vi "AalborgDFCCommand.vi"(4 "Channel Name":string="Aalborg", 6 "Port Name":string="mfc1", 7 "Timeout/ms":u32=1500, 8 "Numeric Value":dbl format="%.2f", 9 "AalborgDFCCommand":T2="FullScaleRatingSLPM", 10 "Address":u8 format="%.0x") -> (0 "String Reply":string="!11,100.0000\r\n", 1 "Error Description":string, 2 "Numeric Reply":dbl=100.0, 3 "OK":bool)   [LabVIEW 2016]
uses:
  AalborgDFCCommand.ctl
  AalborgDFCCommandDescriptor.ctl
  AalborgDFCCommandPhases.ctl
panel:
  out "commandString":string
  out "Audit trail":string[](array[string])
  out "CommandDescriptorOutput":T1={"Command"="FullScaleRatingSLPM", "Mnemonic"="E", "Min"=nan, "Max"=nan, "ActionPath"=["PassCommand", "Communicate", "ParseNumber", "Done"]}
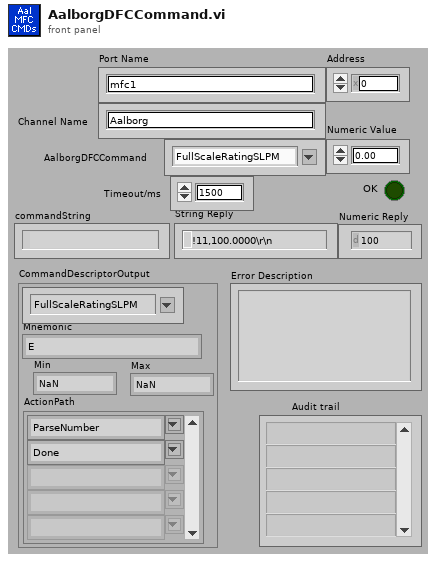
[diagram p1: front panel]
types:
  T1 = typedef "AalborgDFCCommandDescriptor.ctl" = cluster{"Command":T2, "Mnemonic":string, "Min":dbl, "Max":dbl, "ActionPath":T3[]}
  T2 = typedef "AalborgDFCCommand.ctl" = string
  T3 = typedef "AalborgDFCCommandPhases.ctl" = string
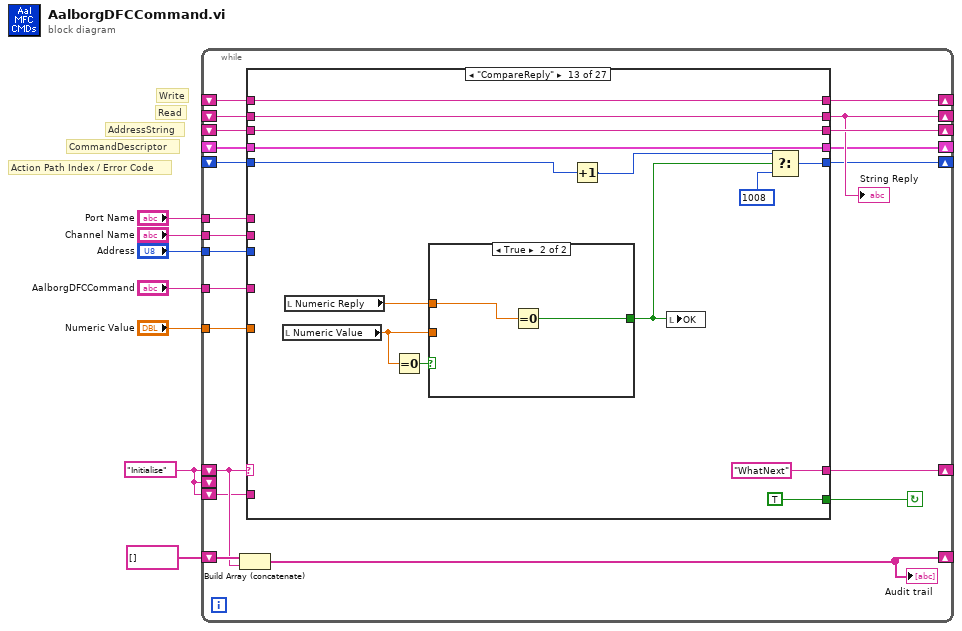
[diagram p0: block diagram]
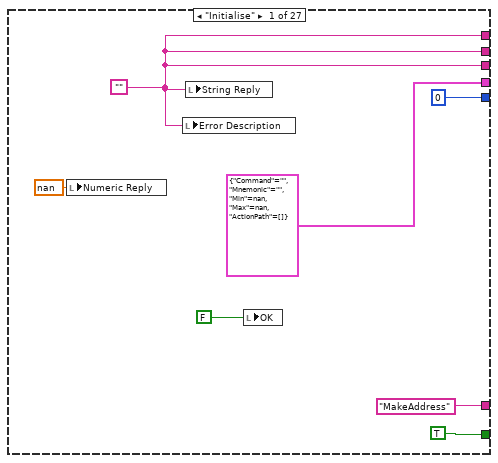
[diagram p2: hidden frame]
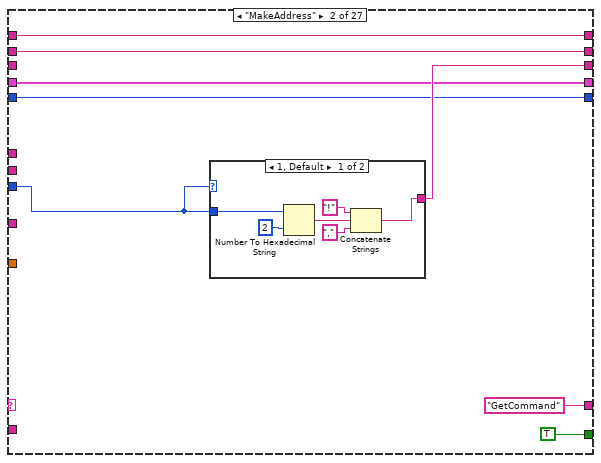
[diagram p3: hidden frame]
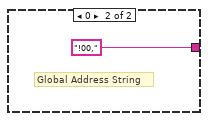
[diagram p4: hidden frame]
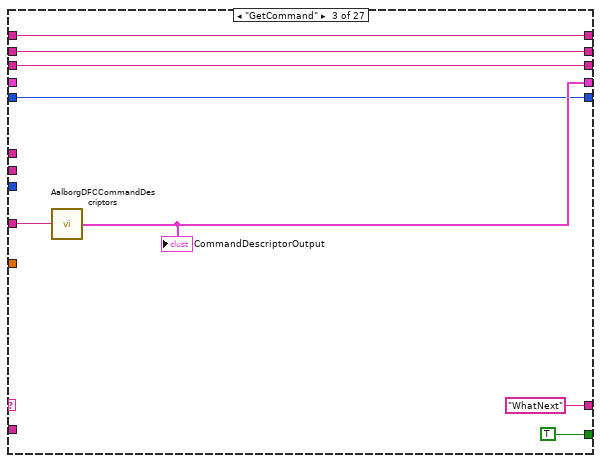
[diagram p5: hidden frame]
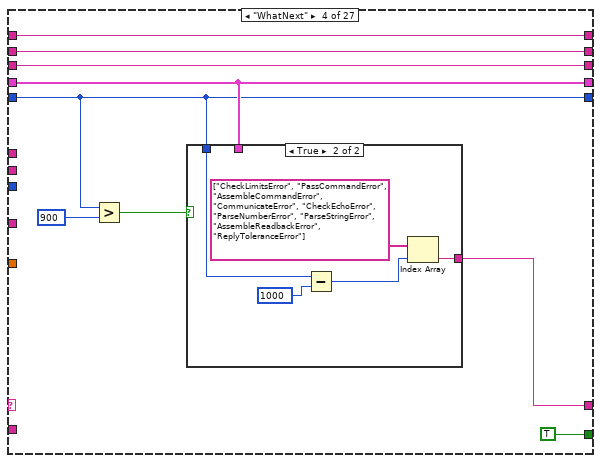
[diagram p6: hidden frame]
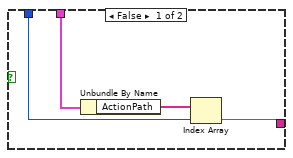
[diagram p7: hidden frame]
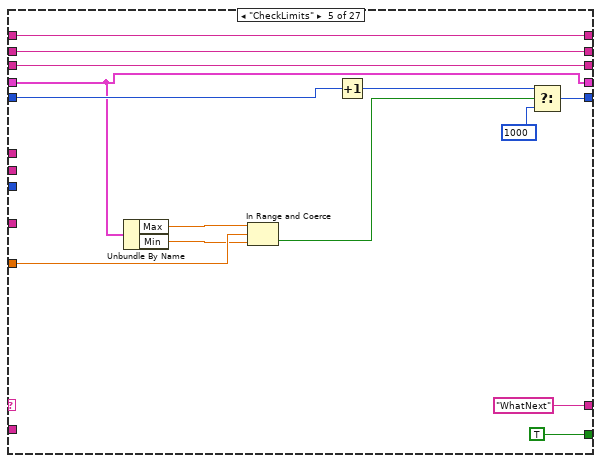
[diagram p8: hidden frame]
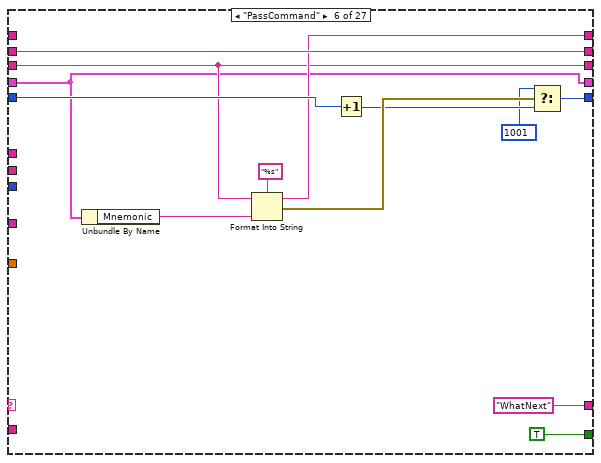
[diagram p9: hidden frame]
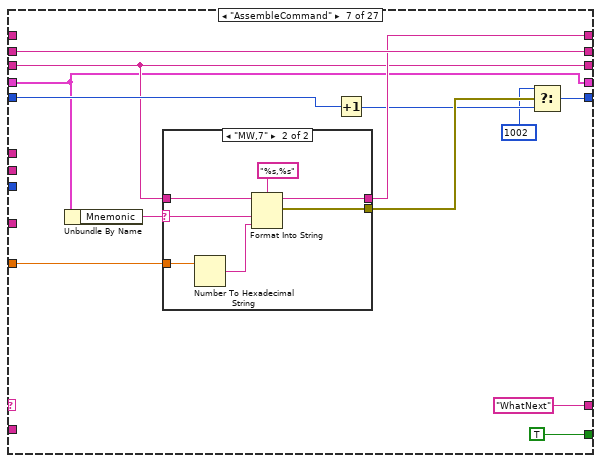
[diagram p10: hidden frame]
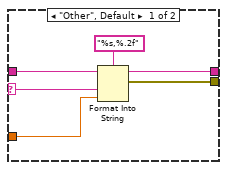
[diagram p11: hidden frame]
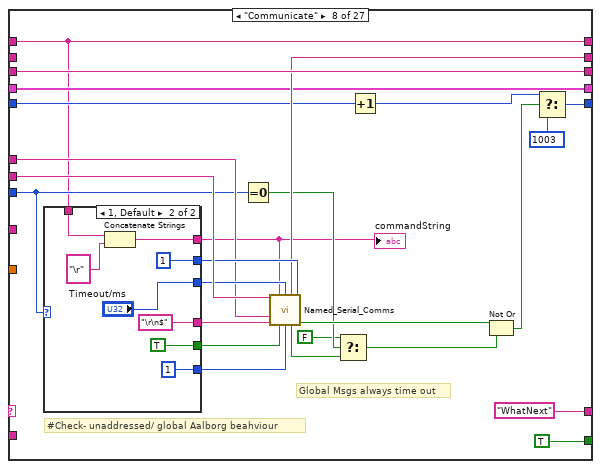
[diagram p12: hidden frame]
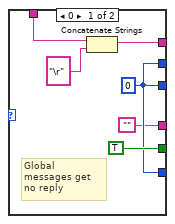
[diagram p13: hidden frame]
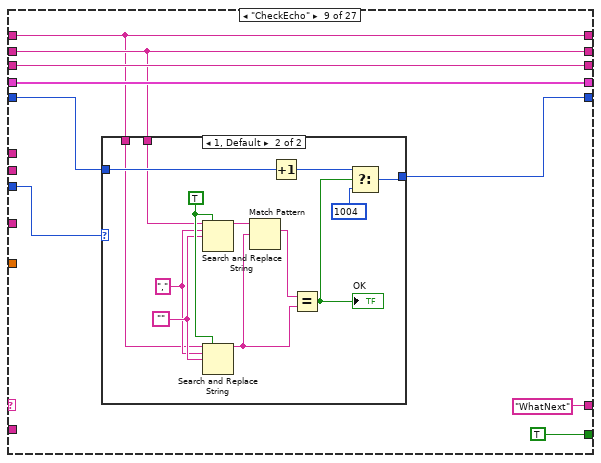
[diagram p14: hidden frame]
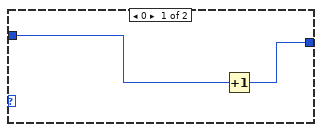
[diagram p15: hidden frame]
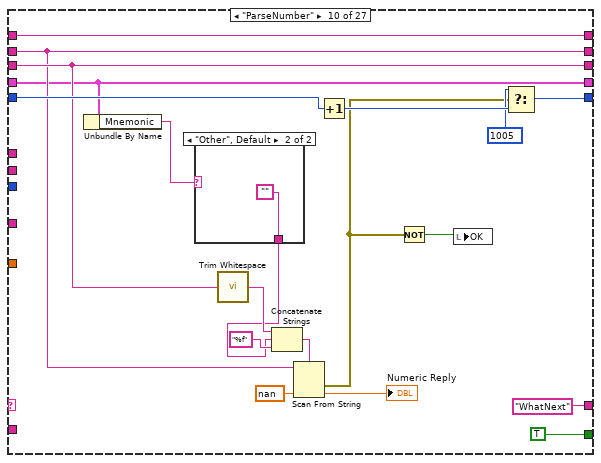
[diagram p16: hidden frame]
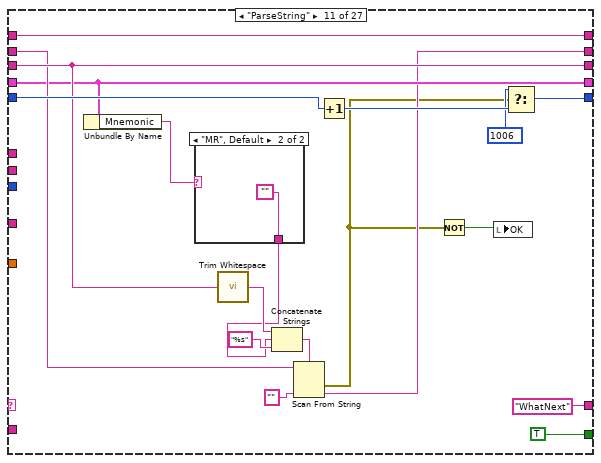
[diagram p18: hidden frame]
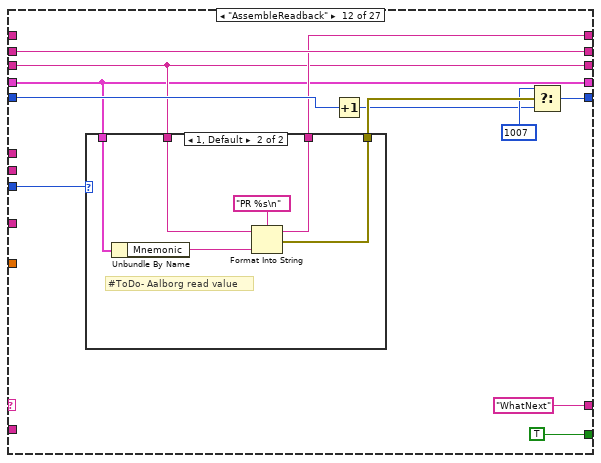
[diagram p20: hidden frame]
diagram:
  w1 = "Initialise"
  # "Action Path Index / Error Code"
  # "CommandDescriptor"
  # "AddressString"
  # "Read"
  # "Write"
  n1 = while {
    shift-right: [w16] -> _
    shift-left: w1 -> [w10]
    tunnel: "Address" -> [w28]
    tunnel: "AalborgDFCCommand" -> [w27]
    tunnel: "Numeric Value" -> [w26]
    shift-right: [w25] -> _
    shift-left: _ -> [w24]
    tunnel: "Port Name" -> [w23]
    tunnel: "Channel Name" -> [w22]
    shift-right: [w15] -> _
    shift-left: _ -> [w21]
    shift-right: [w19] -> _
    shift-left: _ -> [w18]
    shift-right: [w8] -> _
    shift-left: string[] [] -> [w17]
    shift-right: [w14] -> _
    shift-left: _ -> [w13]
    shift-right: [w11] -> _
    shift-left: _ -> [w12]
    shift-left: w1 -> [_]
    shift-left: w1 -> [w9]
    stop <- w20 continue-if-true
    n2 = Build Array (concatenate)(w17, w10) -> (w8:T3[])
    "Audit trail" <- w8
    n3 = case shown="\"CompareReply\"" w10 {
      selector: w10 -> [_ _ _ _ _ _ _ _ _ _ _ _ _ _ _ _ _ _ _ _ _ _ _ _ _ _ w445]
      tunnel: ["MakeAddress" "GetCommand" "WhatNext" w63 "WhatNext" "WhatNext" "WhatNext" "WhatNext" "WhatNext" "WhatNext" "WhatNext" "WhatNext" "WhatNext" w281 "Error" "Initialise" "Error" "Error" "Error" "Error" "Error" "Error" "Error" "Error" "Error" "Error" w445] -> w16
      tunnel: w28 -> [_ w36 _ _ _ _ _ w132 w169 _ _ w238 _ _ _ _ w333 w344 w354 w365 w375 w387 w399 w410 w421 w430 _]
      tunnel: w27 -> [_ _ w55 _ _ _ _ _ _ _ _ _ _ _ _ _ _ _ _ _ _ _ _ _ _ _ _]
      tunnel: w26 -> [_ _ _ _ w88 _ w105 _ _ _ _ _ _ _ _ _ w336 _ w357 _ _ _ _ _ _ _ _]
      tunnel: [w30 w41 w57 w66 w86 w98 w111 w131 w170 w200 w223 w241 w261 w287 w303 w331 w341 w351 w362 w372 w384 w396 w407 w418 w427 w438 w443] -> w25
      tunnel: w24 -> [_ w41 w57 w66 w86 _ _ w131 w170 w200 w223 _ w261 w287 w303 w324 _ _ _ _ w378 w390 _ _ _ _ _]
      tunnel: w23 -> [_ _ _ _ _ _ _ w148 _ _ _ _ _ _ _ w325 _ _ _ _ _ _ _ _ _ _ _]
      tunnel: w22 -> [_ _ _ _ _ _ _ w154 _ _ _ _ _ _ w298 w326 _ _ _ _ _ _ _ _ _ _ _]
      tunnel: [w30 w40 w56 w65 w90 w103 w116 w145 w171 w198 w216 w246 w268 w285 w308 w331 w341 w351 w362 w372 w384 w396 w407 w418 w427 w438 w443] -> w15
      tunnel: w21 -> [_ w40 w56 w65 w90 w103 w116 _ w171 w198 w221 w246 w268 w285 w308 w323 _ _ _ _ w377 w389 w401 w412 _ w432 _]
      tunnel: [TRUE TRUE ("Continue") TRUE ("Continue") TRUE ("Continue") TRUE TRUE TRUE TRUE TRUE TRUE TRUE TRUE TRUE w282 TRUE w315 TRUE ("Continue") TRUE ("Continue") TRUE ("Continue") TRUE ("Continue") TRUE ("Continue") TRUE ("Continue") TRUE ("Continue") TRUE ("Continue") TRUE ("Continue") TRUE ("Continue") FALSE] -> w20
      tunnel: [w30 w43 w54 w64 w89 w97 w110 w146 w176 w199 w222 w239 w263 w286 w313 w331 w341 w351 w362 w372 w384 w396 w407 w418 w427 w438 w443] -> w19
      tunnel: w18 -> [_ _ w54 w64 w89 w97 w110 w146 w176 w199 w222 w239 w263 w286 w313 _ _ _ _ _ _ _ _ _ _ _ _]
      tunnel: [T1 {"Command"="", "Mnemonic"="", "Min"=nan, "Max"=nan, "ActionPath"=[]} ("CommandDescriptorOutput") w38 w52 w62 w77 w94 w109 w144 w172 w197 w220 w237 w262 w279 w309 w330 w339 w349 w360 w370 w382 w394 w405 w416 w425 w436 w442] -> w14
      tunnel: w13 -> [_ w38 _ w62 w77 w94 w109 w144 w172 w197 w220 w237 w262 w278 w309 w330 w339 w349 w360 w370 w382 w394 w405 w416 w425 w436 w442]
      tunnel: w12 -> [_ w37 w51 w61 w81 w99 w112 w139 w173 w208 w229 w242 w264 _ w310 w329 w340 w350 w361 w371 w383 w395 w406 w417 w426 w437 w441]
      tunnel: [0 w37 w51 w61 w82 w100 w113 w141 w174 w209 w230 w243 w265 0 ("f") w311 w329 w340 w350 w361 w371 w383 w395 w406 w417 w426 w437 w441] -> w11
      tunnel: w9 -> [_ _ _ _ _ _ _ _ _ _ _ _ _ _ _ w321 _ _ _ _ _ _ _ _ _ _ _]
      frame "Initialise" {
        w30 = ""
        n4 = local write "Numeric Reply"(nan ("Numeric Reply")) -> ()
        n5 = local write "Error Description"(w30) -> ()
        n6 = local write "String Reply"(w30) -> ()
        n7 = local write "OK"(FALSE ("GoodEcho")) -> ()
      }
      frame "MakeAddress" {
        n8 = case shown="1, Default" w36 {
          tunnel: w36 -> [w44 _]
          tunnel: [w45 "!00,"] -> w43
          frame 1, Default {
            n9 = Number To Hexadecimal String(1:i16 2 ("width (-)"), 2:w44) -> (0:w48:string)
            n10 = Concatenate Strings("!" ("string"), w48, "," ("string")) -> (w45:string)
          }
          frame 0 {
            # "Global Address String"
          }
        }
      }
      frame "GetCommand" {
        n11 = call "AalborgDFCCommandDescriptors.vi"("AalborgDFCCommand"=w55) -> ("CommandDescriptorOutput"=w52:T1)  [unwired: 4 out]
        "CommandDescriptorOutput" <- w52
      }
      frame "WhatNext" {
        n12 = Greater?(x=w61, y=900) -> (0:w59:bool)
        n13 = case shown="True" w59 {
          tunnel: [w70 w72] -> w63
          tunnel: w62 -> [w69 _]
          tunnel: w61 -> [w68 w75]
          frame False {
            n14 = Unbundle By Name(w69) -> ("ActionPath"=w71:T3[])
            n15 = Index Array(array=w71, index=w68) -> (element=w70:T3)
          }
          frame True {
            n16 = Subtract(x=w75, y=1000) -> (x-y=w73:i32)
            n17 = Index Array(array=string[] ["CheckLimitsError", "PassCommandError", "AssembleCommandError", "CommunicateError", "CheckEchoError", "ParseNumberError", "ParseStringError", "AssembleReadbackError", "ReplyToleranceError"], index=w73) -> (element=w72:string)
          }
        }
      }
      frame "CheckLimits" {
        n18 = Unbundle By Name(w77) -> ("Max"=w85:dbl, "Min"=w84:dbl)
        n19 = In Range and Coerce(upper limit=w85, x=w88, lower limit=w84) -> (In Range?=w79:bool)  [unwired: 1 out]
        n20 = Increment(x=w81) -> (x+1=w80:i32)
        n21 = Select(t=w80, s=w79, f=1000) -> (s? t:f=w82:i32)
      }
      frame "PassCommand" {
        n22 = Unbundle By Name(w94) -> ("Mnemonic"=w96:string)
        n23 = Format Into String(format string="%s", initial string=w97, w96) -> (resulting string=w98:string, error out=w93:errorcluster)  [unwired: 1 in]
        n24 = Increment(x=w99) -> (x+1=w92:i32)
        n25 = Select(t=1001 ("f"), s=w93, f=w92) -> (s? t:f=w100:i32)
      }
      frame "AssembleCommand" {
        n26 = Unbundle By Name(w109) -> ("Mnemonic"=w104:string)
        n27 = case shown="\"MW,7\"" w104 {
          selector: w104 -> [w117 w123]
          tunnel: [w122 w129] -> w111
          tunnel: w110 -> [w121 w128]
          tunnel: [w119 w126] -> w108
          tunnel: w105 -> [w118 w125]
          frame "Other", Default {
            n28 = Format Into String(format string="%s,%.2f", initial string=w121, w117, w118) -> (resulting string=w122:string, error out=w119:errorcluster)  [unwired: 1 in]
          }
          frame "MW,7" {
            n29 = Number To Hexadecimal String(2:w125) -> (0:w124:string)  [unwired: 1 in]
            n30 = Format Into String(format string="%s,%s", initial string=w128, w123, w124) -> (resulting string=w129:string, error out=w126:errorcluster)  [unwired: 1 in]
          }
        }
        n31 = Increment(x=w112) -> (x+1=w107:i32)
        n32 = Select(t=1002 ("f"), s=w108, f=w107) -> (s? t:f=w113:i32)
      }
      frame "Communicate" {
        # "#Check- unaddressed/ global Aalborg beahviour"
        # "Global Msgs always time out"
        n33 = case shown="1, Default" w132 {
          tunnel: ["" "\r\n$"] -> w153
          tunnel: [w159 1 ("Terminate Count")] -> w152
          tunnel: [w159 "Timeout/ms"] -> w151
          tunnel: [TRUE ("Log Errors?") TRUE ("Log Errors?")] -> w150
          tunnel: [w159 1 ("!Error retries")] -> w149
          tunnel: w131 -> [w156 w163]
          tunnel: [w157 w162] -> w130
          frame 0 {
            w159 = 0 ("!Error retries")
            # "Global messages get no reply"
            n34 = Concatenate Strings(w156, "\r" ("string")) -> (w157:string)
          }
          frame 1, Default {
            n35 = Concatenate Strings(w163, "\r" ("string")) -> (w162:string)
          }
        }
        "commandString" <- w130
        n36 = Equal To 0?(x=w132) -> (x = 0?=w135:bool)
        n37 = call "Named_Serial_Comms.vi"("Channel Name"=w154, "Write"=w130, "Timeout/ms"=w151, "!Error retries"=w149, "Port Name"=w148, "Term Grep"=w153, "Log Errors?"=w150, "Terminate Count"=w152) -> ("Read"=w145:string, "Timed out"=w134:bool, "Serial Error"=w142:bool)  [unwired: 1 in, 4 out]
        n38 = Select(t=FALSE, s=w135, f=w134) -> (s? t:f=w136:bool)
        n39 = Increment(x=w139) -> (x+1=w138:i32)
        n40 = Not Or(1:w136, 2:w142) -> (0:w140:bool)
        n41 = Select(t=w138, s=w140, f=1003) -> (s? t:f=w141:i32)
      }
      frame "CheckEcho" {
        n42 = case shown="1, Default" w169 {
          tunnel: [w178 w191] -> w174
          tunnel: w173 -> [w179 w189]
          tunnel: w171 -> [_ w182]
          tunnel: w170 -> [_ w181]
          frame 0 {
            n43 = Increment(x=w179) -> (x+1=w178:i32)
          }
          frame 1, Default {
            w183 = "," ("search string")
            w188 = TRUE ("replace all? (F)")
            w187 = ""
            n44 = Search and Replace String(replace all?=w188, input string=w182, search string=w183, replace string=w187) -> (result string=w186:string)  [unwired: 4 in, 3 out]
            n45 = Search and Replace String(replace all?=w188, input string=w181, search string=w183, replace string=w187) -> (result string=w184:string)  [unwired: 4 in, 3 out]
            n46 = Match Pattern(string=w186, regular expression=w184) -> (match substring=w185:string)  [unwired: 1 in, 3 out]
            n47 = Increment(x=w189) -> (x+1=w190:i32)
            n48 = Equal?(x=w185, y=w184) -> (x = y?=w180:bool)
            "OK" <- w180
            n49 = Select(t=w190, s=w180, f=1004) -> (s? t:f=w191:i32)
          }
        }
      }
      frame "ParseNumber" {
        n50 = Unbundle By Name(w197) -> ("Mnemonic"=w196:string)
        n51 = case shown="\"Other\", Default" w196 {
          selector: w196 -> [w212 _]
          tunnel: [w212 ""] -> w195
          frame "S" {
          }
          frame "Other", Default {
          }
        }
        n52 = call <vilib>:"Trim Whitespace.vi"("string"=w199) -> ("trimmed string"=w201:string)  [unwired: 1 in]
        n53 = Concatenate Strings(w201, w195, "%f" ("format string")) -> (w203:string)
        n54 = Scan From String(format string=w203, input string=w198, default 1=nan ("default value 1")) -> (error out=w194:errorcluster, output 1=→"Numeric Reply":dbl)  [unwired: 2 in, 2 out]
        n55 = Increment(x=w208) -> (x+1=w206:i32)
        n56 = Not(x=w194) -> (.not. x?=w193:bool)
        n57 = local write "OK"(w193) -> ()
        n58 = Select(t=1005, s=w194, f=w206) -> (s? t:f=w209:i32)
      }
      frame "ParseString" {
        n59 = Unbundle By Name(w220) -> ("Mnemonic"=w219:string)
        n60 = case shown="\"MR\", Default" w219 {
          selector: w219 -> [w233 _]
          tunnel: [w233 ""] -> w218
          frame "MW" {
          }
          frame "MR", Default {
          }
        }
        n61 = call <vilib>:"Trim Whitespace.vi"("string"=w222) -> ("trimmed string"=w224:string)  [unwired: 1 in]
        n62 = Concatenate Strings(w224, w218, "%s" ("format string")) -> (w226:string)
        n63 = Scan From String(format string=w226, input string=w221, default 1="") -> (error out=w214:errorcluster, output 1=w216:string)  [unwired: 2 in, 2 out]
        n64 = Increment(x=w229) -> (x+1=w228:i32)
        n65 = Not(x=w214) -> (.not. x?=w215:bool)
        n66 = local write "OK"(w215) -> ()
        n67 = Select(t=1006, s=w214, f=w228) -> (s? t:f=w230:i32)
      }
      frame "AssembleReadback" {
        n68 = case shown="1, Default" w238 {
          tunnel: w237 -> [_ w254]
          tunnel: ["" w253] -> w241
          tunnel: [errorcluster {"status"=TRUE, "code"=0, "source"=""} ("error IO") w252] -> w240
          tunnel: w239 -> [_ w251]
          frame 0 {
            # "Can't READ globally..."
          }
          frame 1, Default {
            # "#ToDo- Aalborg read value"
            n69 = Unbundle By Name(w254) -> ("Mnemonic"=w250:string)
            n70 = Format Into String(format string="PR %s\n", initial string=w251, w250) -> (resulting string=w253:string, error out=w252:errorcluster)  [unwired: 1 in]
          }
        }
        n71 = Increment(x=w242) -> (x+1=w235:i32)
        n72 = Select(t=1007 ("f"), s=w240, f=w235) -> (s? t:f=w243:i32)
      }
      frame "CompareReply" {
        n73 = local read "Numeric Value"() -> (w255:dbl)
        n74 = local read "Numeric Reply"() -> (w260:dbl)
        n75 = Equal To 0?(x=w255) -> (x = 0?=w256:bool)
        n76 = case shown="True" w256 {
          tunnel: w260 -> [w275 w277]
          tunnel: w255 -> [w272 _]
          tunnel: [w269 w276] -> w257
          frame False {
            n77 = Subtract(x=w275, y=w272) -> (x-y=w274:dbl)
            n78 = Absolute Value(x=w274) -> (abs(x)=w273:dbl)
            n79 = Divide(x=w273, y=w272) -> (x/y=w271:dbl)
            n80 = Less?(x=w271, y=0.001) -> (x < y?=w269:bool)
          }
          frame True {
            n81 = Equal To 0?(x=w277) -> (x = 0?=w276:bool)
          }
        }
        n82 = Increment(x=w264) -> (x+1=w258:i32)
        n83 = local write "OK"(w257) -> ()
        n84 = Select(t=w258, s=w257, f=1008) -> (s? t:f=w265:i32)
      }
      frame "Done" {
        # "#Check- What is the error prompt from Aalborgs?"
        n85 = Match Pattern(string=w285, regular expression="?") -> (offset past match=w280:i32)  [unwired: 4 out]
        n86 = case shown="0, Default" w280 {
          tunnel: [TRUE ("Continue") FALSE ("Continue")] -> w282
          tunnel: ["WhatNext" "Initialise"] -> w281
          tunnel: [w291 w292] -> w279
          tunnel: w278 -> [_ w292]
          frame 0, Default {
            # "#Check- What should we do \nif there's an error?"
            n87 = call "AalborgDFCCommandDescriptors.vi"("AalborgDFCCommand"=T2 "ValveStatus") -> ("CommandDescriptorOutput"=w291:T1)  [unwired: 4 out]
          }
          frame -1 {
          }
        }
      }
      frame "ParseError" {
        n88 = call <vilib>:"Trim Whitespace.vi"("string"=w303) -> ("trimmed string"=w301:string)  [unwired: 1 in]
        n89 = Concatenate Strings(w301, "%s" ("format string")) -> (w304:string)
        n90 = Scan From String(format string=w304, input string=w308, default 1="") -> (error out=w307:errorcluster, output 1=w299:string)  [unwired: 2 in, 2 out]
        n91 = call "AalborgDFCErrorCodes.vi"("Error Code"=w299) -> ("Error Description"=w297:string)  [unwired: 4 out]
        n92 = Increment(x=w310) -> (x+1=w306:i32)
        n93 = Format Into String(format string="The %s has %s", w298, w297) -> (resulting string=→"Error Description":string)  [unwired: 2 in, 1 out]
        n94 = Select(t=1007, s=w307, f=w306) -> (s? t:f=w311:i32)
      }
      frame "Error" {
        w318 = "Error in AalborgDFCCommand.vi: " ("string")
        w331 = ""
        w315 = FALSE ("Continue")
        n95 = local read "Error Description"() -> (w317:string)
        n96 = call "Serial_log_build.vi"("Read"=w323, "Write String"=w324, "Port Name"=w325) -> ("Output Array"=w327:string[])
        n97 = Empty String/Path?(string/path=w317) -> (empty?=w322:bool)
        n98 = Concatenate Strings(w318, w321) -> (w320:string)
        n99 = Concatenate Strings(w318, w317) -> (w319:string)
        n100 = Select(t=w320, s=w322, f=w319) -> (s? t:f=w316:string)
        n101 = call "Write_serial_log.vi"("Log Type"="AalborgDFC_Error_Log", "Log Array"=w327, "Header message"=w316, "Channel Name"=w326) -> ()  [unwired: 1 out]
        n102 = local write "OK"(w315) -> ()
      }
      frame "CheckLimitsError" {
        w341 = ""
        n103 = Unbundle By Name(w339) -> ("Mnemonic"=w337:string)
        n104 = Format Into String(format string="%s=%d) to MFC %x", initial string="Attempt to Write an out-of-range value (" ("message"), w337, w336, w333) -> (resulting string=w334:string)  [unwired: 1 in, 1 out]
        n105 = local write "Error Description"(w334) -> ()
      }
      frame "PassCommandError" {
        w351 = ""
        n106 = Unbundle By Name(w349) -> ("Mnemonic"=w347:string)
        n107 = Format Into String(format string="%s) to MFC %x", initial string="Attempt to PassCommand (" ("message"), w347, w344) -> (resulting string=w345:string)  [unwired: 1 in, 1 out]
        n108 = local write "Error Description"(w345) -> ()
      }
      frame "AssembleCommandError" {
        w362 = ""
        n109 = Unbundle By Name(w360) -> ("Mnemonic"=w358:string)
        n110 = Format Into String(format string="%s,%.1f) to MFC %x", initial string="Attempt to AssembleCommand (" ("message"), w358, w357, w354) -> (resulting string=w355:string)  [unwired: 1 in, 1 out]
        n111 = local write "Error Description"(w355) -> ()
      }
      frame "CommunicateError" {
        w372 = ""
        n112 = Unbundle By Name(w370) -> ("Command"=w368:T2)
        n113 = Format Into String(format string="%s) to MFC %x", initial string="Serial CommsError (" ("message"), w368, w365) -> (resulting string=w366:string)  [unwired: 1 in, 1 out]
        n114 = local write "Error Description"(w366) -> ()
      }
      frame "CheckEchoError" {
        w384 = ""
        n115 = Unbundle By Name(w382) -> ("Command"=w380:T2)
        n116 = Format Into String(format string="Command = %s; Write = %s; Read=%s) to MFC %x", initial string="Echo Error (" ("message"), w380, w378, w377, w375) -> (resulting string=w376:string)  [unwired: 1 in, 1 out]
        n117 = local write "Error Description"(w376) -> ()
      }
      frame "ReplyToleranceError" {
        w396 = ""
        n118 = Unbundle By Name(w394) -> ("Command"=w392:T2)
        n119 = Format Into String(format string="Command = %s; Write = %s; Read=%s) to MFC %x", initial string="Reply out of tolerance (" ("message"), w392, w390, w389, w387) -> (resulting string=w388:string)  [unwired: 1 in, 1 out]
        n120 = local write "Error Description"(w388) -> ()
      }
      frame "ParseNumberError" {
        w407 = ""
        n121 = Unbundle By Name(w405) -> ("Mnemonic"=w403:string)
        n122 = Format Into String(format string="%s=%s) from MFC %x", initial string="Attempt to ParseNumber (" ("message"), w403, w401, w399) -> (resulting string=w400:string)  [unwired: 1 in, 1 out]
        n123 = local write "Error Description"(w400) -> ()
      }
      frame "ParseStringError" {
        w418 = ""
        n124 = Unbundle By Name(w416) -> ("Mnemonic"=w414:string)
        n125 = Format Into String(format string="%s=%s) from MFC %x", initial string="Attempt to ParseString (" ("message"), w414, w412, w410) -> (resulting string=w411:string)  [unwired: 1 in, 1 out]
        n126 = local write "Error Description"(w411) -> ()
      }
      frame "AssembleReadbackError" {
        w427 = ""
        n127 = Format Into String(format string="to MFC %x", initial string="Attempt to AssembleReadback " ("message"), w421) -> (resulting string=w422:string)  [unwired: 1 in, 1 out]
        n128 = local write "Error Description"(w422) -> ()
      }
      frame "ParseErrorError" {
        w438 = ""
        n129 = Unbundle By Name(w436) -> ("Command"=w434:T2)
        n130 = Format Into String(format string="Command = %s; Read = %s) for MFC %x", initial string="Attempt to ParseError (" ("message"), w434, w432, w430) -> (resulting string=w431:string)  [unwired: 1 in, 1 out]
        n131 = local write "Error Description"(w431) -> ()
      }
      frame "NoMatch", Default {
        w443 = ""
        n132 = One Button Dialog(message="Case not found in AalborgDFCDriveCommand.vi", button name ("OK")="Shit!...") -> ()  [unwired: 1 out]
      }
    }
    "String Reply" <- w15
  }
